vi "gwyscan preview.vi"(0 "xypos":dbl[](array[numeric]), 1 "zdata":dbl[](array[numeric]), 2 "n":i32, 3 "channel":i32, 4 "preview_image":dbl[](array[numeric]), 5 "preview_mask":dbl[](array[numeric]), 6 "preview_width":i32, 7 "error in (no error)":errorcluster, 8 "preview_height":i32, 9 "preview_xreal":dbl, 10 "preview_yreal":dbl, 11 "preview_xoffset":dbl, 12 "preview_yoffset":dbl, 13 "preview_angle":dbl) -> (22 "function return":i32, 25 "Preview_image":dbl[](array[numeric]), 26 "preview_mask 2":dbl[](array[numeric]), 27 "error out":errorcluster)   [LabVIEW 2016, in "libgwyscan.lvlib"]
doc: "GWYSCANDLL_API int gwyscan_preview(double *xypos, double *zdata, int n, int offset, int channel, double *preview_image, double *preview_mask, int preview_width, int preview_height, double preview_xreal, double preview_yreal, double preview_xoffset, double preview_yoffset, double preview_angle);\n\nGWYSCANDLL_API GwyscanResult gwyscan_preview(const double *xypos, const double *zdata, int n, int channel, double *preview_image, double *preview_mask, int preview_width, int preview_height, double preview_xreal, double preview_yreal, double preview_xoffset, double preview_yoffset, double preview_angle);"
uses:
  libgwyscan.lvlib
  libgwyscan.dll
panel:
  out "zdata":dbl[](array[numeric])
  out "xypos":dbl[](array[numeric])
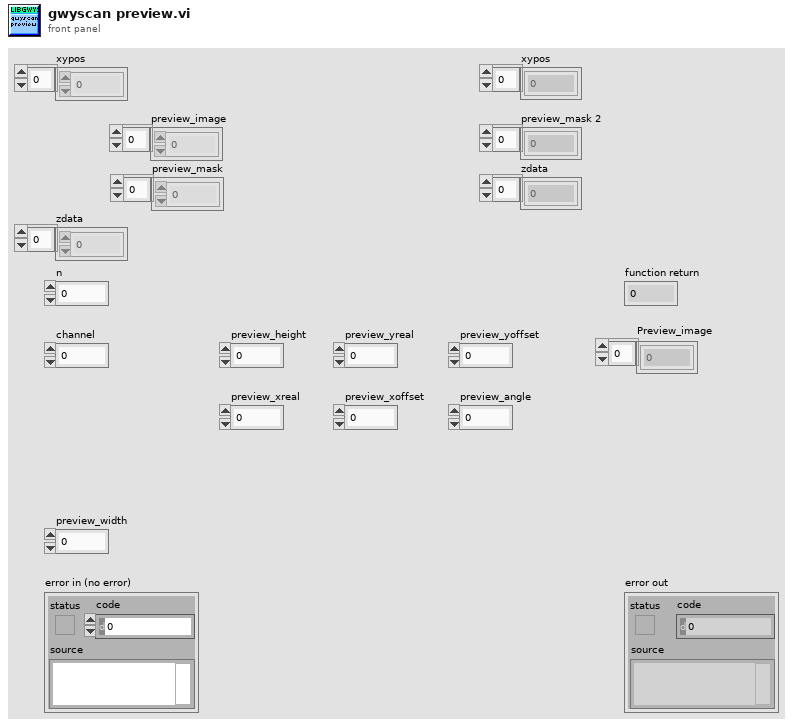
[diagram p1: front panel]
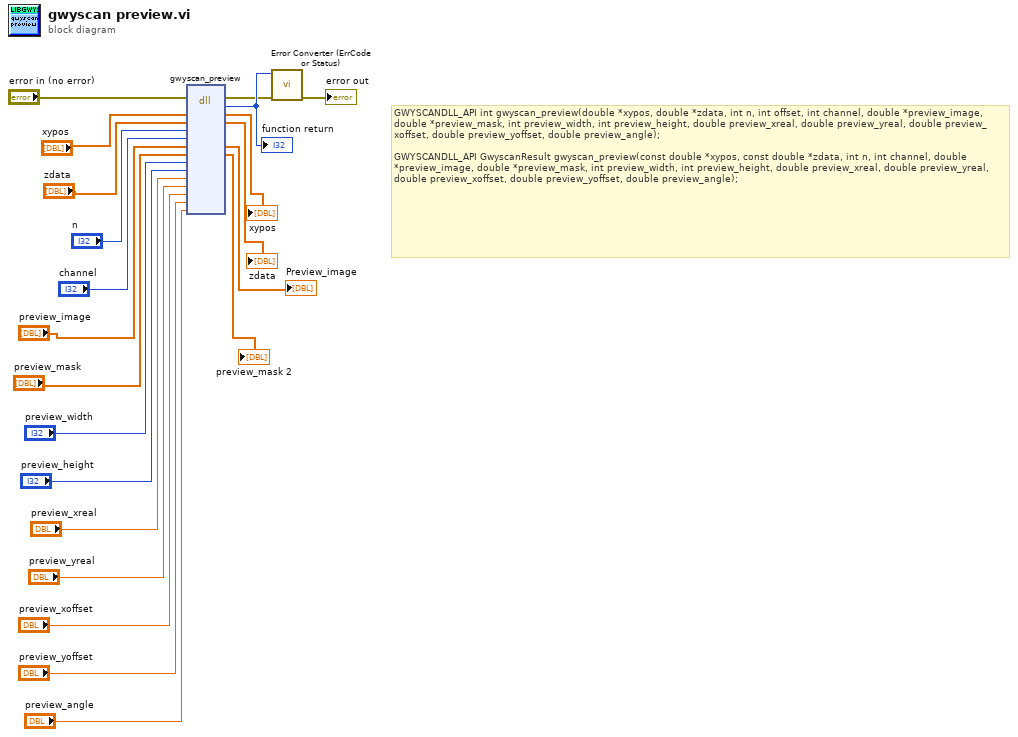
[diagram p0: block diagram]
diagram:
  # "GWYSCANDLL_API int gwyscan_preview(double *xypos, double *zdata, int n, int offset, int channel, double *preview_image, double *preview_mask, int preview_width, int preview_height, double preview_xreal, double preview_yreal, double preview_xoffset, double preview_yoffset, double preview_angle);\n\nGWYSCANDLL_API GwyscanResult gwyscan_preview(const double *xypos, const double *zdata, int n, int channel, double *preview_image, double *preview_mask, int preview_width, int preview_height, double preview_xreal, double preview_yreal, double preview_xoffset, double preview_yoffset, double preview_angle);"
  n1 = dll-call lib="PTH2abs CUsersCharlÃ¨ne BrillardDesktoplbni-lbniAFMController-BetaVersionv2.0.16-20190611 libgwyscan-1.2-labview2015-win32libgwyscan.*" fn="gwyscan_preview"(error in="error in (no error)", "xypos"="xypos", "zdata"="zdata", "n"="n", "channel"="channel", "preview_image"="preview_image", "preview_mask"="preview_mask", "preview_width"="preview_width", "preview_height"="preview_height", "preview_xreal"="preview_xreal", "preview_yreal"="preview_yreal", "preview_xoffset"="preview_xoffset", "preview_yoffset"="preview_yoffset", "preview_angle"="preview_angle") -> (error out=w7:errorcluster, "return type"=w21:i32, "xypos"=→"xypos":dbl[], "zdata"=→"zdata":dbl[], "preview_image"=→"Preview_image":dbl[], "preview_mask"=→"preview_mask 2":dbl[])  [unwired: 11 in, 1 out]
  "function return" <- w21
  n2 = call "Error Converter (ErrCode or Status).vi"("error in (no error)"=w7, "error code"=w21) -> ("error out"=→"error out":errorcluster)  [unwired: 9 in]
